vi "Read Address.vi"(8 "error in (no error)":errorcluster, 11 "Instrument.KH7008 in":refnum<class "Instrument.KH7008.lvclass">) -> (0 "error out":errorcluster, 2 "Address":string, 3 "Instrument.KH7008 out":refnum<class "Instrument.KH7008.lvclass">)   [LabVIEW 2019, in "Instrument.KH7008.lvclass"]
uses:
  Instrument.KH7008.lvclass
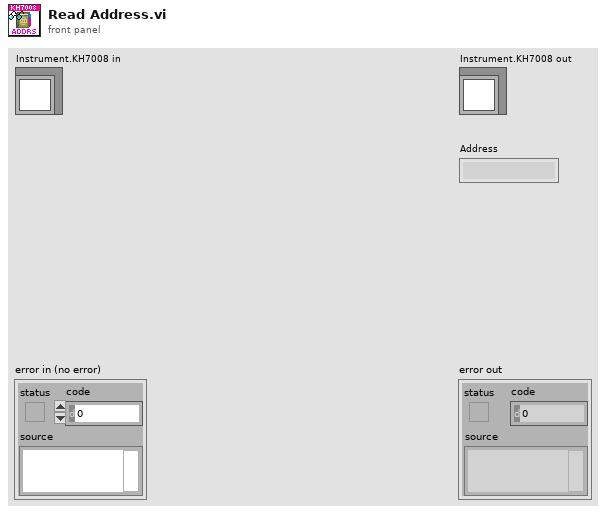
[diagram p1: front panel]
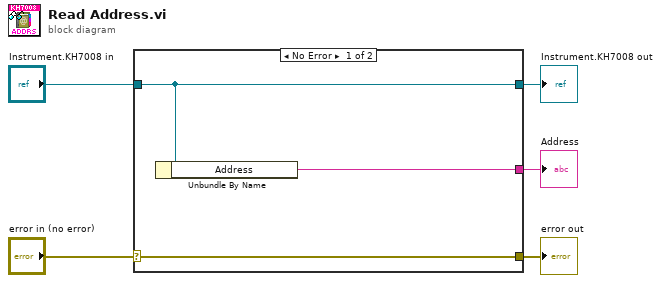
[diagram p0: block diagram]
diagram:
  n1 = case shown="No Error" "error in (no error)" {
    selector: "error in (no error)" -> [w8 w9]
    tunnel: [w8 w9] -> w4
    tunnel: [w7 w10] -> w2
    tunnel: "Instrument.KH7008 in" -> [w7 w10]
    tunnel: [w6 _] -> w1
    frame No Error {
      n2 = Unbundle By Name(w7) -> ("Address"=w6:string)
    }
    frame Error {
    }
  }
  "error out" <- w4
  "Instrument.KH7008 out" <- w2
  "Address" <- w1
